vi "Update ini.vi"(8 "error in (no error)":errorcluster, 11 "Process Settings.lvclass":refnum<class "Process Settings.lvclass">) -> (0 "error out":errorcluster)   [LabVIEW 2017]
uses:
  Process Settings/Process Settings.lvclass
  Process Settings/Process Settings.lvclass/Process Settings.ctl
  Process Settings/Accessors/Read Filename.vi
  <vilib>/Utility/config.llb/Write Key (String).vi
  <vilib>/Utility/config.llb/NI_LVConfig.lvlib
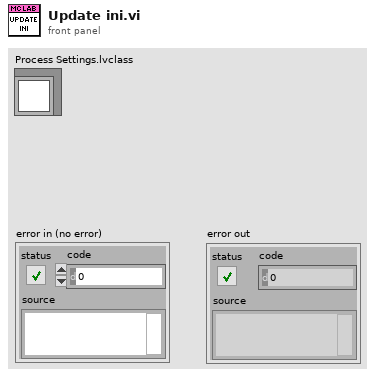
[diagram p1: front panel]
types:
  T1 = typedef "NI_LVConfig.lvlib/Config Data RefNum.ctl" = refnum<k1>
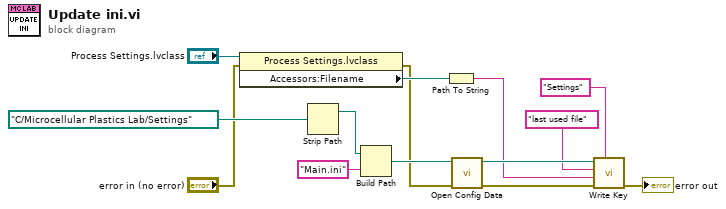
[diagram p0: block diagram]
diagram:
  n1 = property class="Process Settings.lvclass"(reference="Process Settings.lvclass", error in="error in (no error)") -> (error out=w1:errorcluster, "Accessors:Filename"=w4:path)  [unwired: 1 out]
  n2 = Strip Path(path=path "C:/Microcellular Plastics Lab/Settings" ("Path")) -> (stripped path=w13:path)  [unwired: 1 out]
  n3 = Build Path(base path=w13, name or relative path="Main.ini") -> (appended path=w11:path)
  n4 = Path To String(path=w4) -> (string=w3:string)
  n5 = call <vilib>:"Open Config Data.vi"("error in (no error)"=w1, "configuration file path"=w11) -> ("error out"=w9:errorcluster, "refnum"=w10:T1)  [unwired: 7 in, 1 out]
  n6 = call-poly <vilib>:"Write Key.vi"("section"="Settings" ("key"), "error in (no error)"=w9, "value"=w3, "key"="last used file", "refnum"=w10) -> ("error out"=→"error out":errorcluster)  [unwired: 4 in, 2 out]
